vi "05T_Close_connection.vi"(11 "VISA":refnum<visa-resource-name>) -> ()   [LabVIEW 2017]
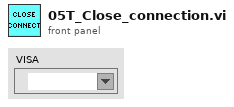
[diagram p1: front panel]
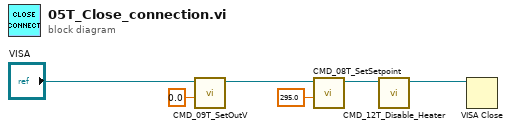
[diagram p0: block diagram]
diagram:
  n1 = call "CMD_09T_SetOutV.vi"("Voltage, d"=0.0, "VISA resource name"="VISA") -> ("VISA resource name out"=w4:refnum<visa-resource-name>)  [unwired: 9 in]
  n2 = call "CMD_08T_SetSetpoint.vi"("Setpoint, K"=295.0, "VISA resource name"=w4) -> ("VISA resource name out"=w3:refnum<visa-resource-name>)  [unwired: 9 in]
  n3 = call "CMD_12T_Disable_Heater.vi"("VISA resource name"=w3) -> ("VISA resource name out"=w2:refnum<visa-resource-name>)  [unwired: 10 in]
  n4 = VISA Close(VISA resource name=w2) -> ()  [unwired: 1 in, 1 out]
